vi "带延迟的多层循环嵌套的反馈节点.vi"() -> ()   [LabVIEW 2020]
panel:
  out "数值":dbl
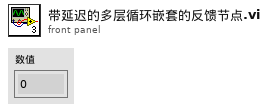
[diagram p1: front panel]
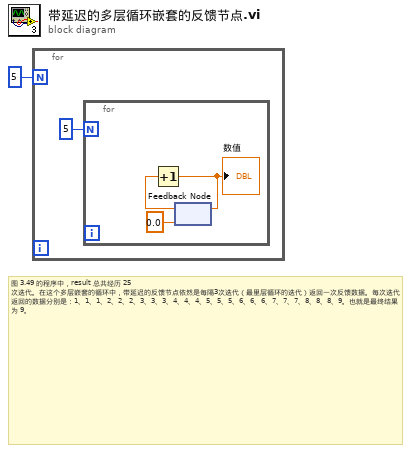
[diagram p0: block diagram]
diagram:
  # "图 3.49 的程序中，result 总共经历 25 次迭代。在这个多层嵌套的循环中，带延迟的反馈节点依然是每隔3次迭代（最里层循环的迭代）返回一次反馈数据。每次迭代返回的数据分别是：1、1、1、2、2、2、3、3、3、4、4、4、5、5、5、6、6、6、7、7、7、8、8、8、9。也就是最终结果为 9。"
  n1 = for {
    N: 5 -> [_]
    n2 = for {
      N: 5 -> [_]
      n3 = feedback #1 ("反馈节点")(0.0) -> (w5:dbl)
      n4 = Increment(x=w5) -> (x+1=w3:dbl)
      "数值" <- w3
      n5 = feedback-in #1(w3) -> ()
    }
  }
